vi "Insert Biometry Data Path.vi"(8 "error in (no error)":errorcluster caption="错误输入（无错误）", 10 "Biometry Data Path":T1, 11 "connection reference":T2) -> (0 "error out":errorcluster caption="错误输出")   [LabVIEW 2015, in "Database Processing.lvlib"]
doc: "该模板用于创建子VI。"
uses:
  Database Processing.lvlib
  <vilib>/addons/database/Connection.llb/Conn ObjectReference.ctl
  Support/Table/Biometry Data Path.ctl
  <vilib>/addons/database/NI_Database_API.lvlib
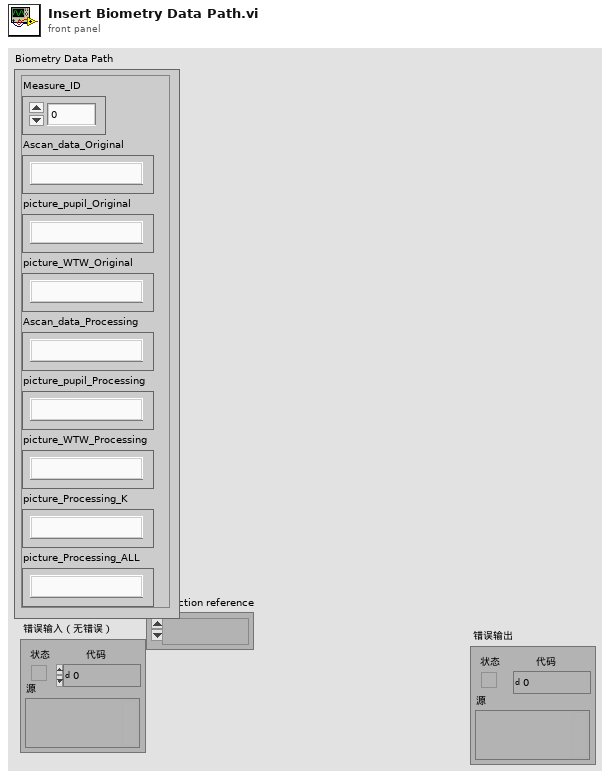
[diagram p1: front panel]
types:
  T1 = typedef "Database Processing.lvlib/Biometry Data Path.ctl" = cluster{"Measure_ID":i64, "Ascan_data_Original":string, "picture_pupil_Original":string, "picture_WTW_Original":string, "Ascan_data_Processing":string, "picture_pupil_Processing":string, "picture_WTW_Processing":string, "picture_Processing_K":string, "picture_Processing_ALL":string}
  T2 = typedef "NI_Database_API.lvlib/Conn ObjectReference.ctl" = refnum<k1>
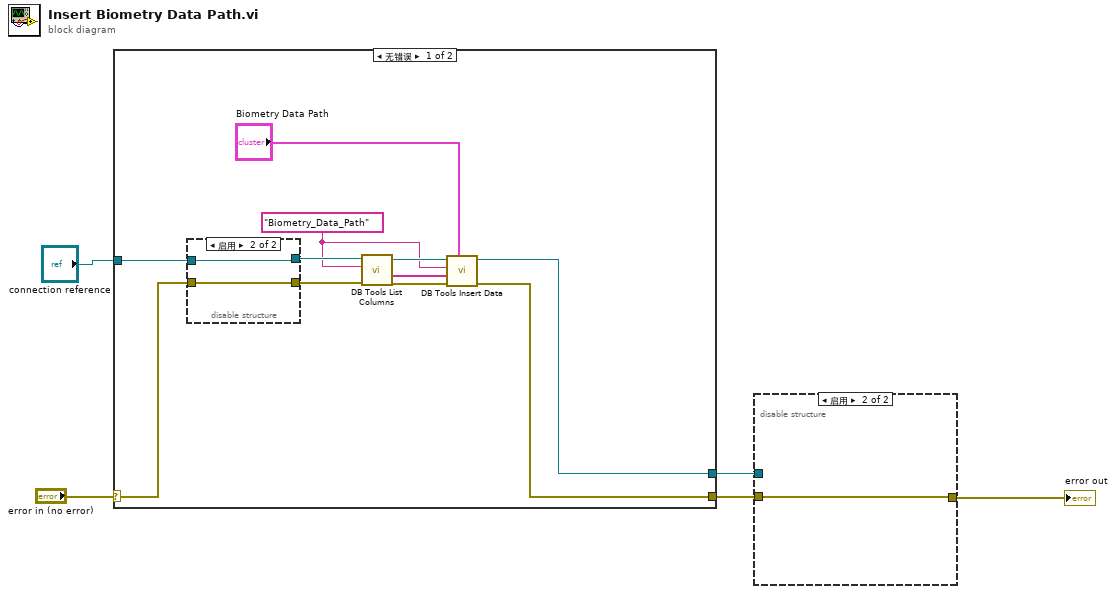
[diagram p0: block diagram]
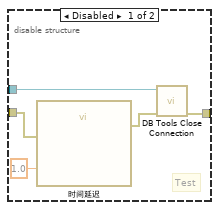
[diagram p2: hidden frame]
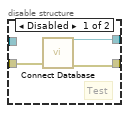
[diagram p3: hidden frame]
diagram:
  n1 = case shown="无错误" "error in (no error)" {
    selector: "error in (no error)" -> [w13 w23]
    tunnel: [w7 w23] -> w2
    tunnel: "connection reference" -> [w15 w22]
    tunnel: [w8 w22] -> w3
    frame No Error {
      w10 = "Biometry_Data_Path" ("table")
      n2 = disable-structure shown="启用" {
        disable-tunnel: [w19 w21] -> w16
        disable-tunnel: w15 -> [_ w21]
        disable-tunnel: w13 -> [w18 w20]
        disable-tunnel: [w17 w20] -> w14
        frame Disabled {
          # "Test"
          n3 = call "Connect Database.vi"("error in (no error)"=w18) -> ("error out"=w17:errorcluster, "connection reference"=w19:T2)  [unwired: 9 in]
        }
        frame Enabled {
        }
      }
      n4 = call <vilib>:"DB Tools List Columns.vi"("error in (no error)"=w14, "table"=w10, "connection reference"=w16) -> ("error out"=w12:errorcluster, "columns"=w9:string[], "connection reference out"=w11:T2)  [unwired: 1 in, 1 out]
      n5 = call <vilib>:"DB Tools Insert Data.vi"("data"="Biometry Data Path", "error in (no error)"=w12, "columns"=w9, "table"=w10, "connection reference"=w11) -> ("error out"=w7:errorcluster, "connection reference out"=w8:T2)  [unwired: 5 in]
    }
    frame Error {
    }
  }
  n6 = disable-structure shown="启用" {
    disable-tunnel: w2 -> [w26 w29]
    disable-tunnel: [w28 w29] -> w1
    disable-tunnel: w3 -> [w27 _]
    frame Disabled {
      # "Test"
      n7 = call "时间延迟"("error in (no error)"=w26, "Delay Time (s)"=1.0) -> ("error out"=w25:errorcluster)  [unwired: 9 in]
      n8 = call <vilib>:"DB Tools Close Connection.vi"("error in (no error)"=w25, "connection reference"=w27) -> ("error out"=w28:errorcluster)  [unwired: 5 in]
    }
    frame Enabled {
    }
  }
  "error out" <- w1
